vi "ResetBEC.vi"(8 "error in (no error)":errorcluster, 11 "board_sel":u32=1) -> (0 "error out":errorcluster)   [LabVIEW 2015, in "ESLSCDLL.lvlib"]
uses:
  ESLSCDLL.lvlib
  ESLSCDLL.dll
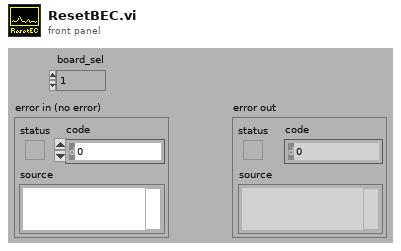
[diagram p1: front panel]
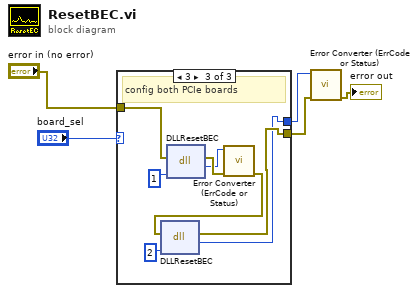
[diagram p0: block diagram]
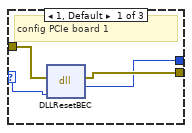
[diagram p2: hidden frame]
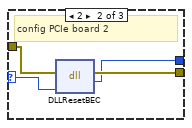
[diagram p3: hidden frame]
diagram:
  n1 = case shown="3" "board_sel" {
    selector: "board_sel" -> [w9 w13 _]
    tunnel: [w7 w12 w15] -> w3
    tunnel: [w6 w11 w14] -> w2
    tunnel: "error in (no error)" -> [w8 w10 w19]
    frame 1, Default {
      # "config PCIe board 1"
      n2 = dll-call lib="C:/Users/flori/Nextcloud/Dokumente/Stresing/Windows/lv64/board.vis/ESLSCDLL.dll" fn="DLLResetBEC" ("lwlscdll.dll:DLLSetTemp")(error in=w8, "drv"=w9) -> (error out=w7:errorcluster, "es_status_codes"=w6:i32)  [unwired: 3 in, 1 out]
    }
    frame 2 {
      # "config PCIe board 2"
      n3 = dll-call lib="C:/Users/flori/Nextcloud/Dokumente/Stresing/Windows/lv64/board.vis/ESLSCDLL.dll" fn="DLLResetBEC" ("lwlscdll.dll:DLLSetTemp")(error in=w10, "drv"=w13) -> (error out=w12:errorcluster, "es_status_codes"=w11:i32)  [unwired: 3 in, 1 out]
    }
    frame 3 {
      # "config both PCIe boards"
      n4 = dll-call lib="C:/Users/flori/Nextcloud/Dokumente/Stresing/Windows/lv64/board.vis/ESLSCDLL.dll" fn="DLLResetBEC" ("lwlscdll.dll:DLLSetTemp")(error in=w19, "drv"=u32 1) -> (error out=w18:errorcluster, "es_status_codes"=w17:i32)  [unwired: 3 in, 1 out]
      n5 = call "Error Converter (ErrCode or Status).vi"("error in (no error)"=w18, "error code"=w17) -> ("error out"=w16:errorcluster)  [unwired: 9 in]
      n6 = dll-call lib="C:/Users/flori/Nextcloud/Dokumente/Stresing/Windows/lv64/board.vis/ESLSCDLL.dll" fn="DLLResetBEC" ("lwlscdll.dll:DLLSetTemp")(error in=w16, "drv"=u32 2) -> (error out=w15:errorcluster, "es_status_codes"=w14:i32)  [unwired: 3 in, 1 out]
    }
  }
  n7 = call "Error Converter (ErrCode or Status).vi"("error in (no error)"=w3, "error code"=w2) -> ("error out"=→"error out":errorcluster)  [unwired: 9 in]
